vi "KH7008 Enum Shunt to Gain.vi"(1 "Shunt Resistor":T1) -> (0 "Gain (V/A)":dbl)   [LabVIEW 2019, in "Inst.Krohn-Hite-7008.lvclass"]
uses:
  Inst.Krohn-Hite-7008.lvclass
  Typedefs/Shunt-Enum.ctl
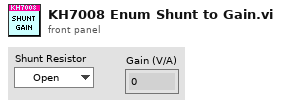
[diagram p1: front panel]
types:
  T1 = typedef "Inst.Krohn-Hite-7008.lvclass/Shunt-Enum.ctl" = enum16{"Open", "50 Ohms", "500 Ohms", "5k Ohms", "50k Ohms", "10M Ohm"}
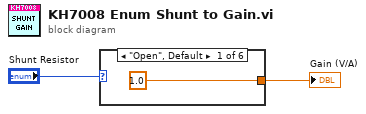
[diagram p0: block diagram]
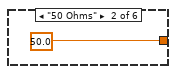
[diagram p2: hidden frame]
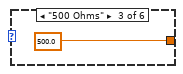
[diagram p3: hidden frame]
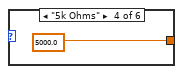
[diagram p4: hidden frame]
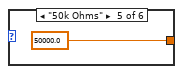
[diagram p5: hidden frame]
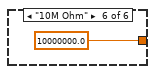
[diagram p6: hidden frame]
diagram:
  n1 = case shown="\"Open\", Default" "Shunt Resistor" {
    tunnel: [1.0 ("y") 50.0 ("y") 500.0 ("y") 5000.0 ("y") 50000.0 ("y") 10000000.0 ("y")] -> w1
    frame "Open", Default {
    }
    frame "50 Ohms" {
    }
    frame "500 Ohms" {
    }
    frame "5k Ohms" {
    }
    frame "50k Ohms" {
    }
    frame "10M Ohm" {
    }
  }
  "Gain (V/A)" <- w1
